vi "GlobalVars.vi"() -> ()   [LabVIEW 2019]
panel:
  out "aux_portlist_0":u16[](array[numeric])
  out "main_portlist_0":u16[](array[numeric])
  out "GBIP0":u32
  out "xt0":u32
  out "aux_portlist":u16[][](array[numeric])
  out "xt end":u32
  out "xt length":u32
  out "GPIBmatrix":string[][](array[string])
  out "main_portlist":u16[][](array[numeric]) format="%0d"
  out "xtlist":u32[](array[numeric])
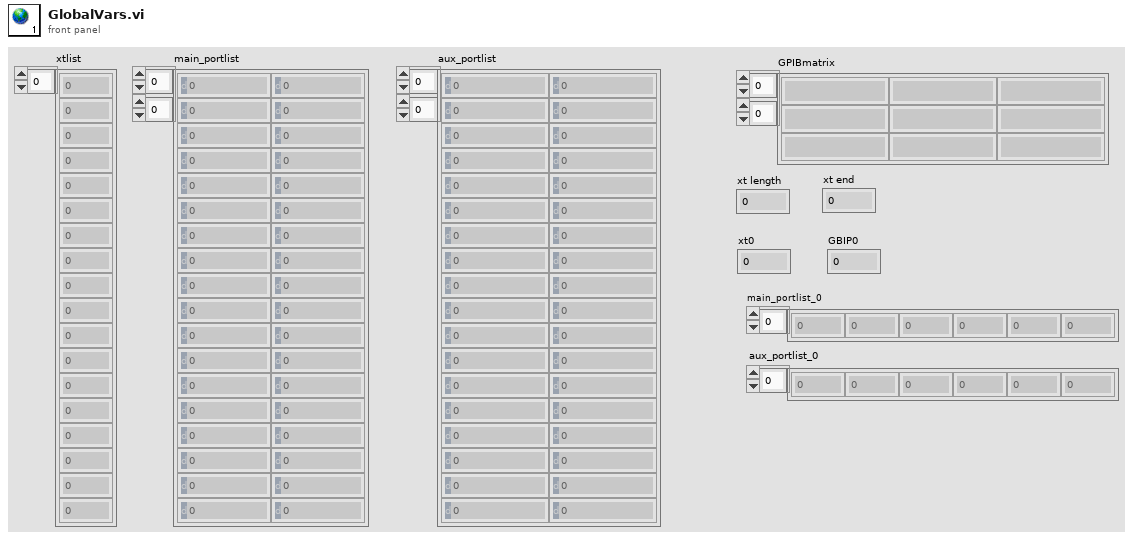
[diagram p1: front panel]
diagram:
